vi "Read Current Measurement.vi"   [LabVIEW 2013, in "California Instruments iX Series.lvlib"]
doc: "Reads single or multiple current measurement(s)."
uses:
  <instrlib>/California Instruments iX Series/California Instruments iX Series.lvlib
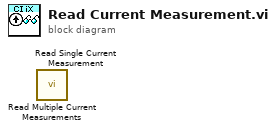
[diagram p0: block diagram]
diagram:
  n1 = call <instrlib>:"Read Multiple Current Measurements.vi"() -> ()  [unwired: 9 in, 3 out]
  n2 = call <instrlib>:"Read Single Current Measurement.vi"() -> ()  [unwired: 9 in, 3 out]
